vi "VI Tree.vi"   [LabVIEW 2010, in "Agilent 33XXX Series.lvlib"]
doc: "This is the instrument driver for the Agilent 33XXX Series. The VI Tree displays all the user-callable VIs of the instrument driver in an organized table."
uses:
  <instrlib>/Agilent 33XXX Series/Agilent 33XXX Series.lvlib
  <instrlib>/Agilent 33XXX Series/Public/Configure/Configure Modulation (Pulse Width).vi
panel:
  # "(c) 2008 National Instruments.  ALL RIGHTS RESERVED."
  # "SEE DIAGRAM\nFOR VI TREE."
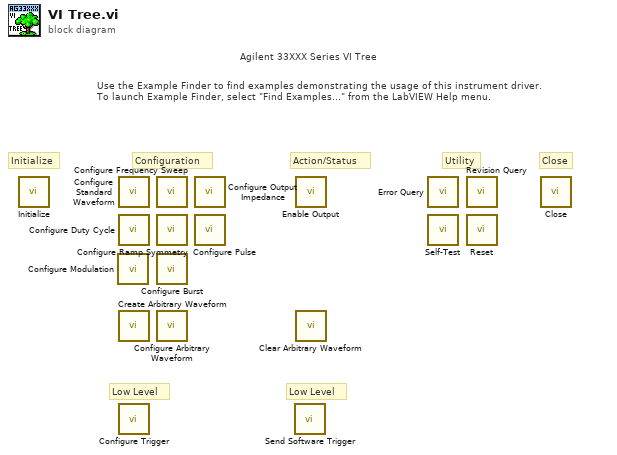
[diagram p0: block diagram]
diagram:
  # "Agilent 33XXX Series VI Tree"
  # "Low Level"
  # "Low Level"
  # "Use the Example Finder to find examples demonstrating the usage of this instrument driver.\nTo launch Example Finder, select \"Find Examples...\" from the LabVIEW Help menu."
  # "Configuration"
  # "Utility"
  # "Action/Status"
  # "Close"
  # "Initialize"
  n1 = call <instrlib>:"Initialize.vi"() -> ()  [unwired: 10 in, 2 out]
  n2 = call-poly <instrlib>:"Configure Modulation.vi"() -> ()  [unwired: 14 in, 2 out]
  n3 = call <instrlib>:"Configure Standard Waveform.vi"() -> ()  [unwired: 10 in, 2 out]
  n4 = call <instrlib>:"Configure Duty Cycle.vi"() -> ()  [unwired: 10 in, 2 out]
  n5 = call <instrlib>:"Create Arbitrary Waveform.vi"() -> ()  [unwired: 10 in, 2 out]
  n6 = call <instrlib>:"Configure Trigger.vi"() -> ()  [unwired: 10 in, 2 out]
  n7 = call <instrlib>:"Configure Frequency Sweep.vi"() -> ()  [unwired: 10 in, 2 out]
  n8 = call <instrlib>:"Configure Ramp Symmetry.vi"() -> ()  [unwired: 10 in, 2 out]
  n9 = call <instrlib>:"Configure Burst.vi"() -> ()  [unwired: 10 in, 2 out]
  n10 = call <instrlib>:"Configure Arbitrary Waveform.vi"() -> ()  [unwired: 10 in, 2 out]
  n11 = call <instrlib>:"Configure Output Impedance.vi"() -> ()  [unwired: 10 in, 2 out]
  n12 = call <instrlib>:"Configure Pulse.vi"() -> ()  [unwired: 10 in, 2 out]
  n13 = call <instrlib>:"Send Software Trigger.vi"() -> ()  [unwired: 10 in, 2 out]
  n14 = call <instrlib>:"Enable Output.vi"() -> ()  [unwired: 10 in, 2 out]
  n15 = call <instrlib>:"Clear Arbitrary Waveform.vi"() -> ()  [unwired: 10 in, 2 out]
  n16 = call <instrlib>:"Error Query.vi"() -> ()  [unwired: 8 in, 4 out]
  n17 = call <instrlib>:"Self-Test.vi"() -> ()  [unwired: 8 in, 4 out]
  n18 = call <instrlib>:"Revision Query.vi"() -> ()  [unwired: 8 in, 4 out]
  n19 = call <instrlib>:"Reset.vi"() -> ()  [unwired: 10 in, 2 out]
  n20 = call <instrlib>:"Close.vi"() -> ()  [unwired: 11 in, 1 out]
